vi "Write Slider Props.vi"(8 "error in (no error)":errorcluster, 10 "Slider Props":T1, 11 "Slider in":refnum<vi>) -> (0 "error out":errorcluster, 3 "Slider":refnum<vi>)   [LabVIEW 2020, in "VolatusGUIEditorCore.lvlib"]
uses:
  VolatusGUIEditorCore.lvlib
  Slider Props.ctl
  Fill Style.ctl
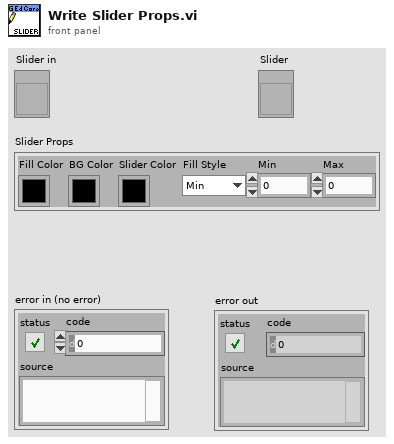
[diagram p1: front panel]
types:
  T1 = typedef "VolatusGUIEditorCore.lvlib/Slider Props.ctl" = cluster{"Fill Color":u32, "BG Color":u32, "Slider Color":u32, "Fill Style":T2, "Min":dbl, "Max":dbl}
  T2 = typedef "VolatusGUIEditorCore.lvlib/Fill Style.ctl" = enum16{"Min", "Max", "None"}
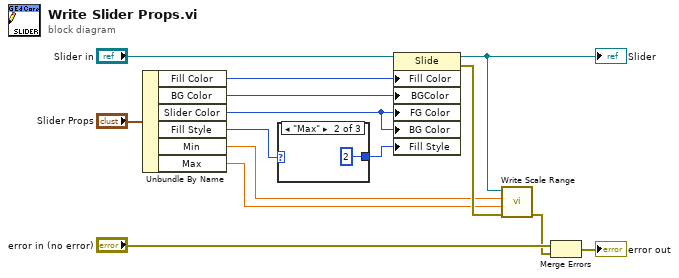
[diagram p0: block diagram]
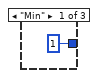
[diagram p2: hidden frame]
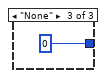
[diagram p3: hidden frame]
diagram:
  n1 = Unbundle By Name("Slider Props") -> ("Fill Color"=w7:u32, "BG Color"=w6:u32, "Slider Color"=w1:u32, "Fill Style"=w3:T2, "Min"=w5:dbl, "Max"=w4:dbl)
  n2 = case shown="\"Max\"" w3 {
    tunnel: [1 2 0] -> w2
    frame "Min" {
    }
    frame "Max" {
    }
    frame "None" {
    }
  }
  n3 = property class="Slide"(reference="Slider in", "Fill Color"=w7, "BGColor"=w6, "FG Color"=w1, "BG Color"=w1, "Fill Style"=w2) -> (reference out=w12:refnum<vi>, error out=w14:errorcluster)  [unwired: 1 in]
  "Slider" <- w12
  n4 = call "Write Scale Range.vi"("error in (no error)"=w14, "Max"=w4, "Min"=w5, "Ctl Refnum in"=w12) -> ("error out"=w10:errorcluster)  [unwired: 6 in, 1 out]
  n5 = Merge Errors("error in (no error)", w10) -> (→"error out":errorcluster)
